vi "Create Row [ ] from Custom Table.vi"(0 "Column Header format":T6, 1 "Header Column size":cluster{"# Column":u16, "# Row":u16}, 2 "Row Header?":bool, 5 "Datas format":T6, 7 "Borders IN":T1, 9 "Row Header format":T6) -> (8 "Row  [ ] OUT":T16)   [LabVIEW 2019]
doc: "Developed by Jean-Marc Simard\nCopyright © 2012, Exaprom Inc.\nAll rights reserved.\nLicense: BSD\n\nWith iTextSharp 4.1.6 (http://itextsharp.sourceforge.net)\nunder Mozilla Public License Version 1.1\n(http://www.mozilla.org/MPL/MPL-1.1.html)"
uses:
  <userlib>/Exaprom PDF/Controls/Table Controls/Table Appearance and Font Row [ ].ctl
  <userlib>/Exaprom PDF/Controls/Table Controls/One Row Appearance.ctl
  <userlib>/Exaprom PDF/Controls/Table Controls/Row from to.ctl
  <userlib>/Exaprom PDF/Controls/Table Controls/Cell, Alignment, LS and Font - hide Vmerge.ctl
  <userlib>/Exaprom PDF/Controls/Table Controls/Cell Type, Alignment and LS.ctl
  <userlib>/Exaprom PDF/Controls/Table Controls/Cell Alignment 20px.ctl
  <userlib>/Exaprom PDF/Controls/Table Controls/Text vertical arrangement.ctl
  <userlib>/Exaprom PDF/Controls/Text Controls/Line spacing.ctl
  <userlib>/Exaprom PDF/Controls/Table Controls/Cell Appearance.ctl
  <userlib>/Exaprom PDF/Controls/Table Controls/Cell Border 20 px.ctl
  <userlib>/Exaprom PDF/Controls/Table Controls/Merge Horizontal.ctl
  <userlib>/Exaprom PDF/Controls/Table Controls/Merge Vertical.ctl
  <userlib>/Exaprom PDF/Controls/Font Controls/Font complete cluster.ctl
  <userlib>/Exaprom PDF/Controls/Font Controls/Font size.ctl
  <userlib>/Exaprom PDF/Controls/Font Controls/Font color.ctl
  <userlib>/Exaprom PDF/Controls/Font Controls/Type and encoding.ctl
  <userlib>/Exaprom PDF/Controls/Text Controls/Unicode/Type and run direction.ctl
  <userlib>/Exaprom PDF/Controls/Table Controls/Cell Font, type, Alignment and LS V2.ctl
  <userlib>/Exaprom PDF/Controls/Table Controls/Simplified Table Row Borders [ ].ctl
  <userlib>/Exaprom PDF/Controls/Table Controls/Simplified Table Row Borders.ctl
  <userlib>/Exaprom PDF/Controls/Table Controls/Border and BG Color [ ].ctl
  <userlib>/Exaprom PDF/Controls/Table Controls/Border and BG Color.ctl
  <userlib>/Exaprom PDF/Controls/Table Controls/Cell, Alignment, LS and Font.ctl
  <userlib>/Exaprom PDF/VIs/Low level/General/Stop if it True.vi
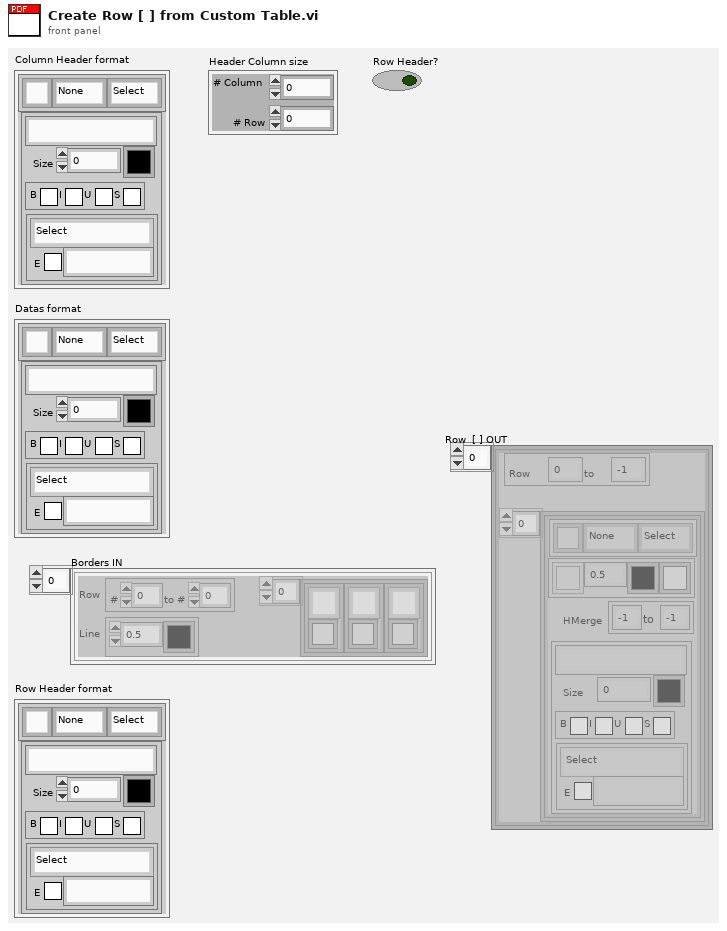
[diagram p1: front panel]
types:
  T1 = typedef "Simplified Table Row Borders [ ].ctl" = T2[]
  T2 = typedef "Simplified Table Row Borders.ctl" = cluster{"Row":cluster{"#":i16, "to #":i16}, "Line":cluster{"Thickness":sgl, "Color":u32}, "Column Borders [ ]":T3}
  T3 = typedef "Border and BG Color [ ].ctl" = T4[]
  T4 = typedef "Border and BG Color.ctl" = cluster{"Cell Border":T5, "BG":u32}
  T5 = typedef "Cell Border 20 px.ctl" = u16
  T6 = typedef "Cell Font, type, Alignment and LS V2.ctl" = cluster{"Cell Type, Alignment and LS":T7, "Font":T11}
  T7 = typedef "Cell Type, Alignment and LS.ctl" = cluster{"Cell Alignment":T8, "Text rotation":T9, "Line spacing":T10}
  T8 = typedef "Cell Alignment 20px.ctl" = u16
  T9 = typedef "Text vertical arrangement.ctl" = enum16{"None", "Clockwise", "Counterclockwise"}
  T10 = typedef "Line spacing.ctl" = enum16{"Select", "1.0", "1.5", "2.0"}
  T11 = typedef "Font complete cluster.ctl" = cluster{"Name":string, "Size":T12, "Color":T13, "Style":cluster{"Bold":bool, "Italic":bool, "Underline":bool, "Strikeout":bool}, "Type":T14}
  T12 = typedef "Font size.ctl" = sgl
  T13 = typedef "Font color.ctl" = u32
  T14 = typedef "Type and encoding.ctl" = cluster{"Type&direction":T15, "Embedded":bool, "Encoding":string}
  T15 = typedef "Type and run direction.ctl" = enum16{"Select", "ASCII", "UTF-16", "UTF-16 (default)", "UTF-16 (LTR)", "UTF-16 (RTL)"}
  T16 = typedef "Table Appearance and Font Row [ ].ctl" = T17[]
  T17 = typedef "One Row Appearance.ctl" = cluster{"Row":T18, "Cell [ ]":T19[]}
  T18 = typedef "Row from to.ctl" = cluster{"From #":i16, "to #":i16}
  T19 = typedef "Cell, Alignment, LS and Font - hide Vmerge.ctl" = cluster{"Text":T7, "Cell Appearance":T20, "HMerge":T21, "VMerge":T22, "Font":T11}
  T20 = typedef "Cell Appearance.ctl" = cluster{"Border":T5, "Thickness":sgl, "Color":u32, "BG":u32}
  T21 = typedef "Merge Horizontal.ctl" = cluster{"From":i8, "to":i8}
  T22 = typedef "Merge Vertical.ctl" = cluster{"From":i8, "to":i8}
  T23 = typedef "Cell, Alignment, LS and Font.ctl" = cluster{"Text":T7, "Cell Appearance":T20, "HMerge":T21, "VMerge":T22, "Font":T11}
  T24 = cluster{"Row":cluster{"#":i16, "to #":i16}, T23[]}
  T25 = cluster{"Row":cluster{"#":i16, "to #":i16}, T23[]}[]
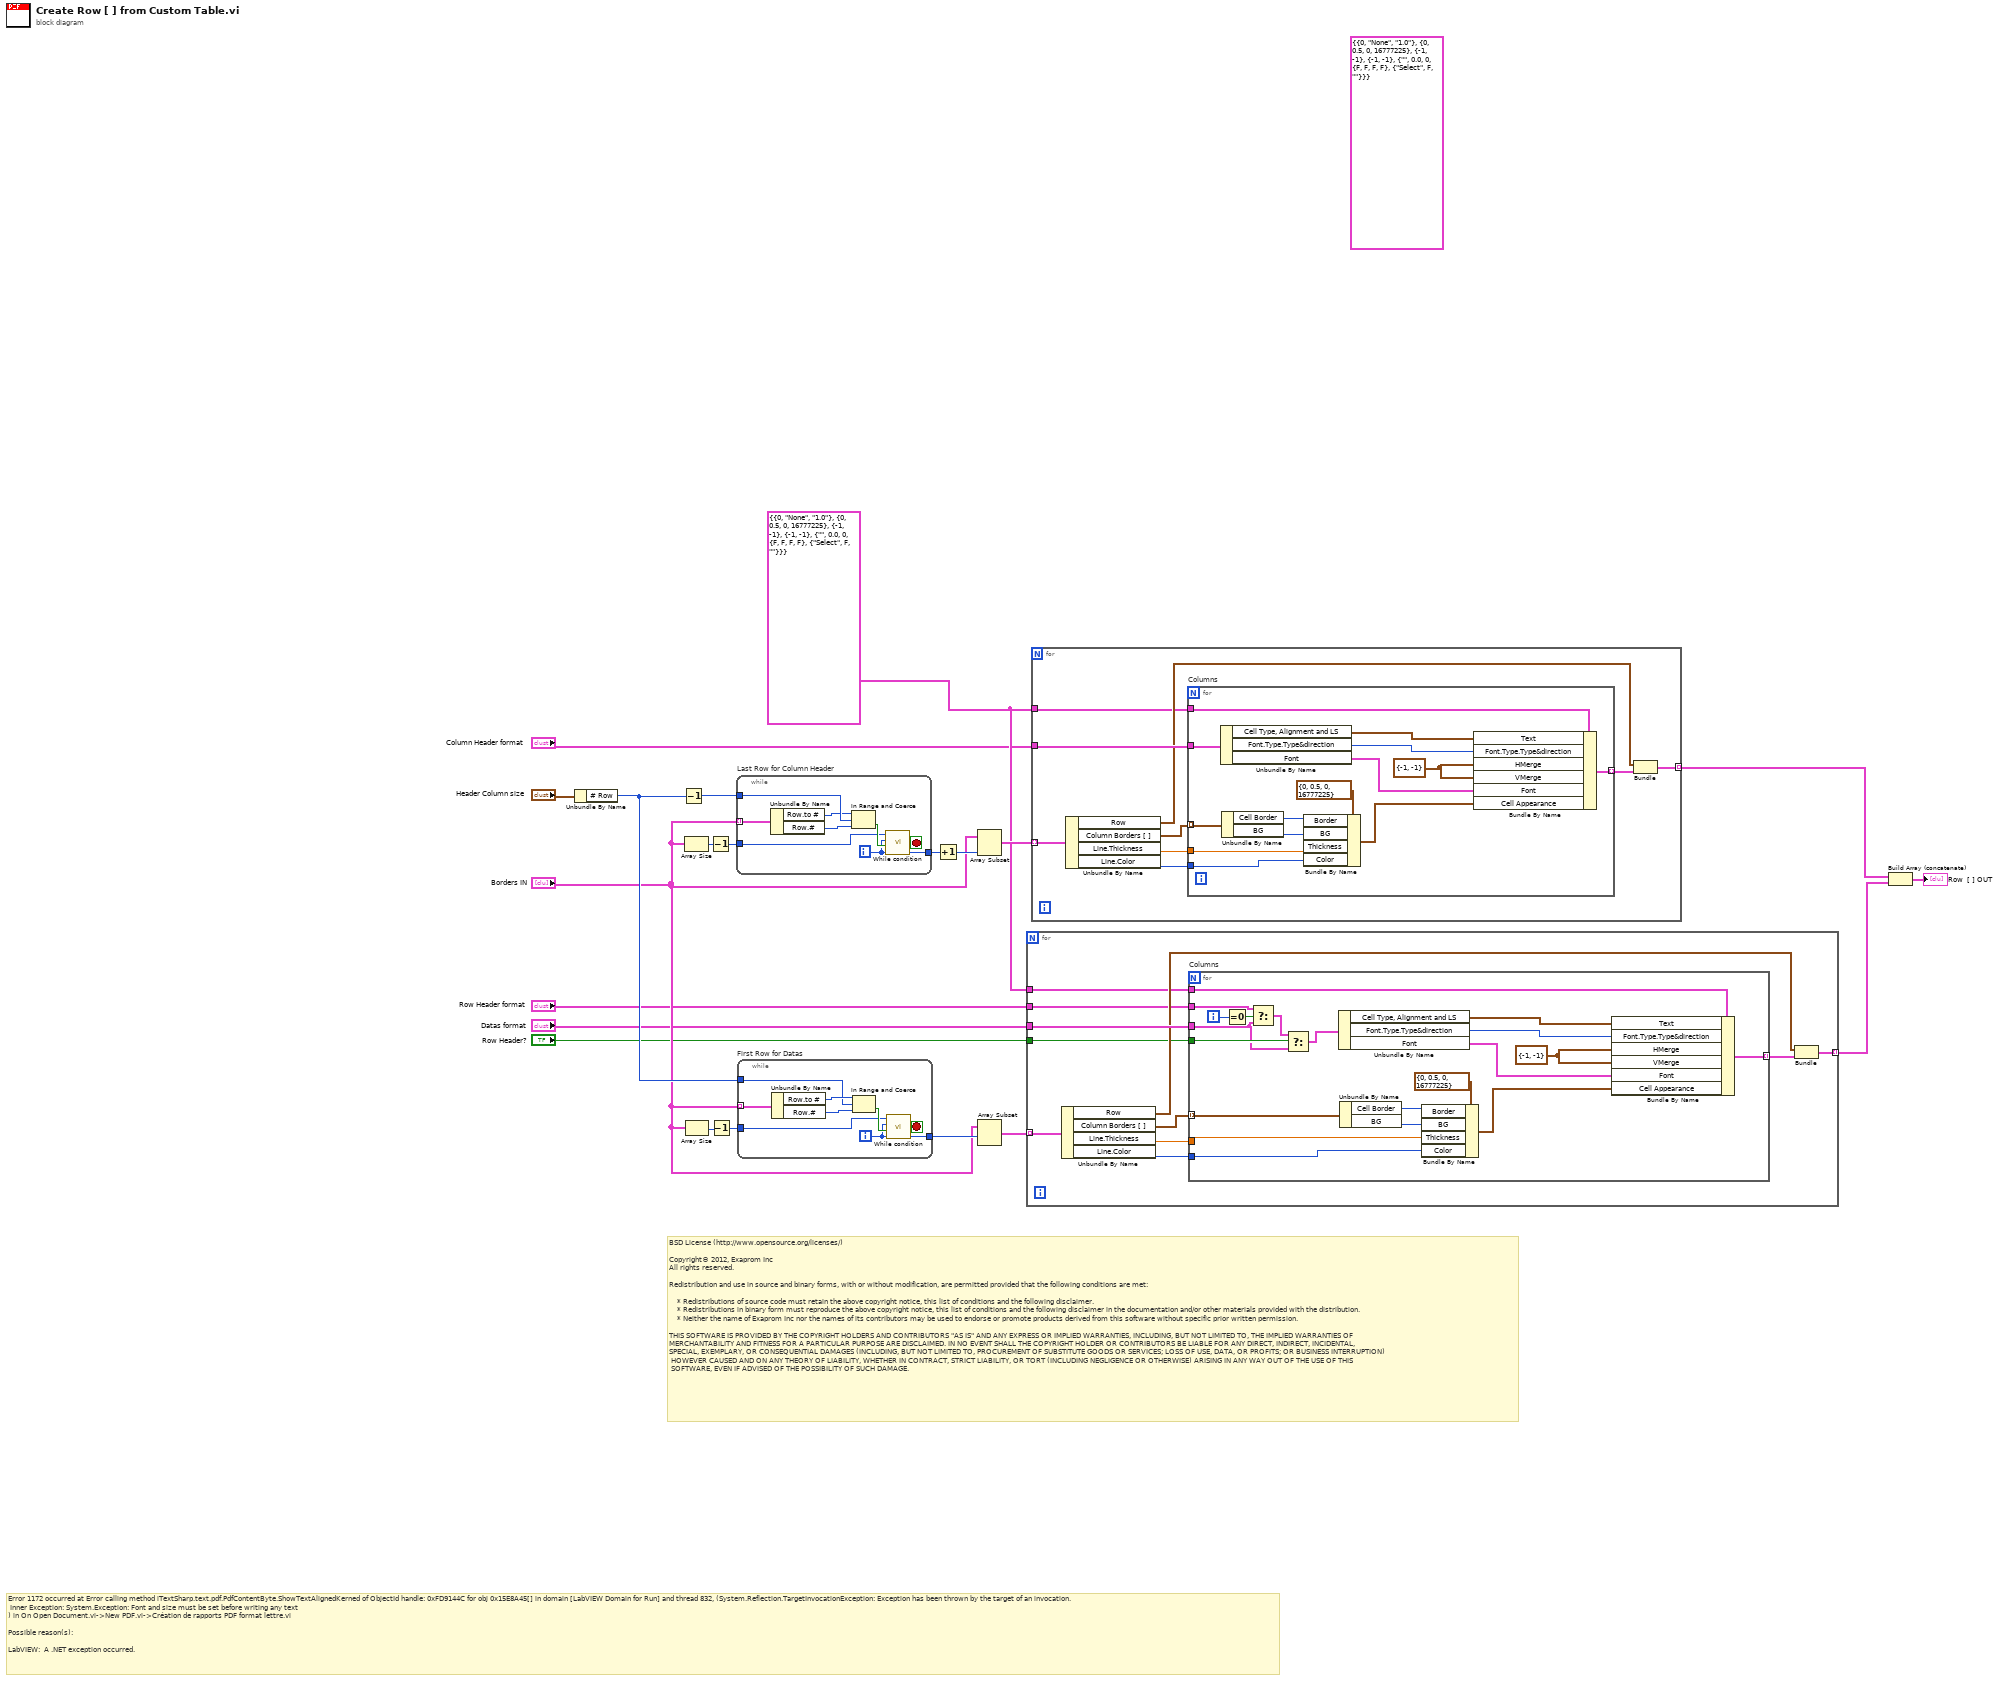
[diagram p0: block diagram]
diagram:
  (unwired) T23 {"Text"={"Cell Alignment"=0, "Text rotation"=enum."None", "Line spacing"=enum."1.0"}, "Cell Appearance"={"Border"=0, "Thickness"=0.5, "Color"=0, "BG"=16777225}, "HMerge"={"From"=-1, "to"=-1}, "VMerge"={"From"=-1, "to"=-1}, "Font"={"Name"="", "Size"=0.0, "Color"=0, "Style"={"Bold"=FALSE, "Italic"=FALSE, "Underline"=FALSE, "Strikeout"=FALSE}, "Type"={"Type&direction"=enum."Select", "Embedded"=FALSE, "Encoding"=""}}} ("Cell, Alignment, LS and Font")
  w8 = T23 {"Text"={"Cell Alignment"=0, "Text rotation"=enum."None", "Line spacing"=enum."1.0"}, "Cell Appearance"={"Border"=0, "Thickness"=0.5, "Color"=0, "BG"=16777225}, "HMerge"={"From"=-1, "to"=-1}, "VMerge"={"From"=-1, "to"=-1}, "Font"={"Name"="", "Size"=0.0, "Color"=0, "Style"={"Bold"=FALSE, "Italic"=FALSE, "Underline"=FALSE, "Strikeout"=FALSE}, "Type"={"Type&direction"=enum."Select", "Embedded"=FALSE, "Encoding"=""}}} ("Cell, Alignment, LS and Font")
  # "Error 1172 occurred at Error calling method iTextSharp.text.pdf.PdfContentByte.ShowTextAlignedKerned of ObjectId handle: 0xFD9144C for obj 0x15E8A45[] in domain [LabVIEW Domain for Run] and thread 832, (System.Reflection.TargetInvocationException: Exception has been thrown by the target of an invocation.\n\tInner Exception: System.Exception: Font and size must be set before writing any text\n) in On Open Document.vi->New PDF.vi->Création de rapports PDF format lettre.vi\n\nPossible reason(s):\n\nLabVIEW:  A .NET exception occurred."
  # "BSD License (http://www.opensource.org/licenses/)\n\nCopyright© 2012, Exaprom Inc\nAll rights reserved.\n\nRedistribution and use in source and binary forms, with or without modification, are permitted provided that the following conditions are met:\n\n    * Redistributions of source code must retain the above copyright notice, this list of conditions and the following disclaimer.\n    * Redistributions in binary form must reproduce the above copyright notice, this list of conditions and the following disclaimer in the documentation and/or other materials provided with the distribution.\n    * Neither the name of Exaprom Inc nor the names of its contributors may be used to endorse or promote products derived from this software without specific prior written permission.\n\nTHIS SOFTWARE IS PROVIDED BY THE COPYRIGHT HOLDERS AND CONTRIBUTORS \"AS IS\" AND ANY EXPRESS OR IMPLIED WARRANTIES, INCLUDING, BUT NOT LIMITED TO, THE IMPLIED WARRANTIES OF \nMERCHANTABILITY AND FITNESS FOR A PARTICULAR PURPOSE ARE DISCLAIMED. IN NO EVENT SHALL THE COPYRIGHT HOLDER OR CONTRIBUTORS BE LIABLE FOR ANY DIRECT, INDIRECT, INCIDENTAL,\nSPECIAL, EXEMPLARY, OR CONSEQUENTIAL DAMAGES (INCLUDING, BUT NOT LIMITED TO, PROCUREMENT OF SUBSTITUTE GOODS OR SERVICES; LOSS OF USE, DATA, OR PROFITS; OR BUSINESS INTERRUPTION)\n HOWEVER CAUSED AND ON ANY THEORY OF LIABILITY, WHETHER IN CONTRACT, STRICT LIABILITY, OR TORT (INCLUDING NEGLIGENCE OR OTHERWISE) ARISING IN ANY WAY OUT OF THE USE OF THIS\n SOFTWARE, EVEN IF ADVISED OF THE POSSIBILITY OF SUCH DAMAGE."
  n1 = Unbundle By Name("Header Column size") -> ("# Row"=w13:u16)
  n2 = Decrement(x=w13) -> (x-1=w14:u16)
  n3 = Array Size(array="Borders IN") -> (size(s)=w20:i32)
  n4 = Array Size(array="Borders IN") -> (size(s)=w16:i32)
  n5 = Decrement(x=w20) -> (x-1=w21:i32)
  n6 = Decrement(x=w16) -> (x-1=w15:i32)
  n7 = while "Last Row for Column Header" {
    tunnel: "Borders IN" -> [w29] mode=indexing
    tunnel: w14 -> [w28]
    tunnel: [w23] -> w18
    tunnel: w21 -> [w22]
    i -> [w23]
    stop <- w25 stop-if-true
    n8 = Unbundle By Name(w29) -> ("Row.to #"=w26:i16, "Row.#"=w27:i16)
    n9 = In Range and Coerce(upper limit=w26, x=w28, lower limit=w27) -> (In Range?=w24:bool)  [unwired: 1 out]
    n10 = call-poly <userlib>:"While condition.vi"("Test"=w24, "i"=w23, "N"=w22) -> ("Action"=w25:bool)  [unwired: 5 out]
  }
  n11 = while "First Row for Datas" {
    tunnel: "Borders IN" -> [w37] mode=indexing
    tunnel: [w32] -> w12
    tunnel: w15 -> [w31]
    tunnel: w13 -> [w30]
    i -> [w32]
    stop <- w34 stop-if-true
    n12 = Unbundle By Name(w37) -> ("Row.to #"=w35:i16, "Row.#"=w36:i16)
    n13 = In Range and Coerce(upper limit=w35, x=w30, lower limit=w36) -> (In Range?=w33:bool)  [unwired: 1 out]
    n14 = call-poly <userlib>:"While condition.vi"("Test"=w33, "i"=w32, "N"=w31) -> ("Action"=w34:bool)  [unwired: 5 out]
  }
  n15 = Increment(x=w18) -> (x+1=w17:i32)
  n16 = Array Subset(array="Borders IN", length=w17) -> (w11:T1)  [unwired: 1 in]
  n17 = Array Subset(array="Borders IN", index=w12) -> (w10:T1)  [unwired: 1 in]
  n18 = for {
    tunnel: w10 -> [w48] mode=indexing
    tunnel: "Datas format" -> [w47]
    tunnel: w8 -> [w41]
    tunnel: [w40] -> w2 mode=indexing
    tunnel: "Row Header format" -> [w39]
    tunnel: "Row Header?" -> [w38]
    n19 = Unbundle By Name(w48) -> ("Row"=w43:cluster{"#":i16, "to #":i16}, "Column Borders [ ]"=w44:T3, "Line.Thickness"=w45:sgl, "Line.Color"=w46:u32)
    n20 = for "Columns" {
      tunnel: w47 -> [w50]
      tunnel: w46 -> [w62]
      tunnel: w45 -> [w61]
      tunnel: w44 -> [w60] mode=indexing
      tunnel: [w57] -> w42 mode=indexing
      tunnel: w41 -> [w56]
      tunnel: w39 -> [w53]
      tunnel: w38 -> [w52]
      i -> [w55]
      w64 = T21 {"From"=-1, "to"=-1} ("HMerge")
      n21 = Equal To 0?(x=w55) -> (x = 0?=w54:bool)
      n22 = Select(t=w53, s=w54, f=w50) -> (s? t:f=w51:T6)
      n23 = Select(t=w51, s=w52, f=w50) -> (s? t:f=w49:T6)
      n24 = Unbundle By Name(w49) -> ("Cell Type, Alignment and LS"=w68:T7, "Font.Type.Type&direction"=w66:T15, "Font"=w63:T11)
      n25 = Unbundle By Name(w60) -> ("Cell Border"=w59:T5, "BG"=w58:u32)
      n26 = Bundle By Name(cluster=T20 {"Border"=0, "Thickness"=0.5, "Color"=0, "BG"=16777225} ("Cell Appearance"), "Border"=w59, "BG"=w58, "Thickness"=w61, "Color"=w62) -> (w65:T20)
      n27 = Bundle By Name(cluster=w56, "Text"=w68, "Font.Type.Type&direction"=w66, "HMerge"=w64, "VMerge"=w64, "Font"=w63, "Cell Appearance"=w65) -> (w57:T23)
    }
    n28 = Bundle("Row"=w43, w42) -> (w40:T24)  [unwired: 1 in]
  }
  n29 = for {
    tunnel: w11 -> [w77] mode=indexing
    tunnel: "Column Header format" -> [w76]
    tunnel: w8 -> [w70]
    tunnel: [w69] -> w3 mode=indexing
    n30 = Unbundle By Name(w77) -> ("Row"=w72:cluster{"#":i16, "to #":i16}, "Column Borders [ ]"=w73:T3, "Line.Thickness"=w74:sgl, "Line.Color"=w75:u32)
    n31 = for "Columns" {
      tunnel: w76 -> [w85]
      tunnel: w75 -> [w84]
      tunnel: w74 -> [w83]
      tunnel: w73 -> [w82] mode=indexing
      tunnel: [w79] -> w71 mode=indexing
      tunnel: w70 -> [w78]
      w87 = T21 {"From"=-1, "to"=-1} ("HMerge")
      n32 = Unbundle By Name(w85) -> ("Cell Type, Alignment and LS"=w91:T7, "Font.Type.Type&direction"=w89:T15, "Font"=w86:T11)
      n33 = Unbundle By Name(w82) -> ("Cell Border"=w81:T5, "BG"=w80:u32)
      n34 = Bundle By Name(cluster=T20 {"Border"=0, "Thickness"=0.5, "Color"=0, "BG"=16777225} ("Cell Appearance"), "Border"=w81, "BG"=w80, "Thickness"=w83, "Color"=w84) -> (w88:T20)
      n35 = Bundle By Name(cluster=w78, "Text"=w91, "Font.Type.Type&direction"=w89, "HMerge"=w87, "VMerge"=w87, "Font"=w86, "Cell Appearance"=w88) -> (w79:T23)
    }
    n36 = Bundle("Row"=w72, w71) -> (w69:T24)  [unwired: 1 in]
  }
  n37 = Build Array (concatenate)(w3, w2) -> (→"Row  [ ] OUT":T25)
